vi "Previous VI.vi"(0 "PDF Report IN":refnum<class "PDF Report Class.lvclass">, 11 "error in (no error)":errorcluster) -> (4 "PDF Report OUT":refnum<class "PDF Report Class.lvclass">, 8 "Execute Actual VI":bool caption="实际执行 VI", 15 "error out":errorcluster)   [LabVIEW 2020, in "Exaprom PDF.lvlib"]
doc: "Version 1.0\nDeveloped by Jean-Marc Simard\nCopyright © 2010, Exaprom Inc.\nAll rights reserved.\nLicense: BSD\n\nWith iTextSharp 4.1.6 (http://itextsharp.sourceforge.net)\nunder Mozilla Public License Version 1.1\n(http://www.mozilla.org/MPL/MPL-1.1.html)"
uses:
  <userlib>/labview-PDF-writer-master/Exaprom PDF.lvlib
  <userlib>/labview-PDF-writer-master/LV Class/PDF Report Class/PDF Report Class.lvclass
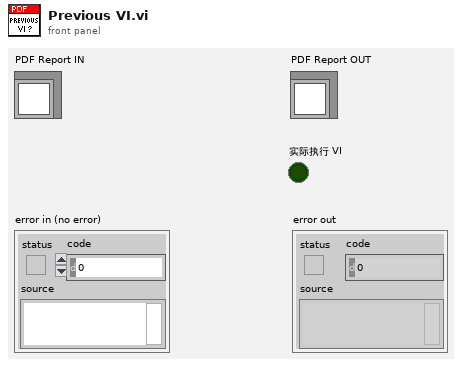
[diagram p1: front panel]
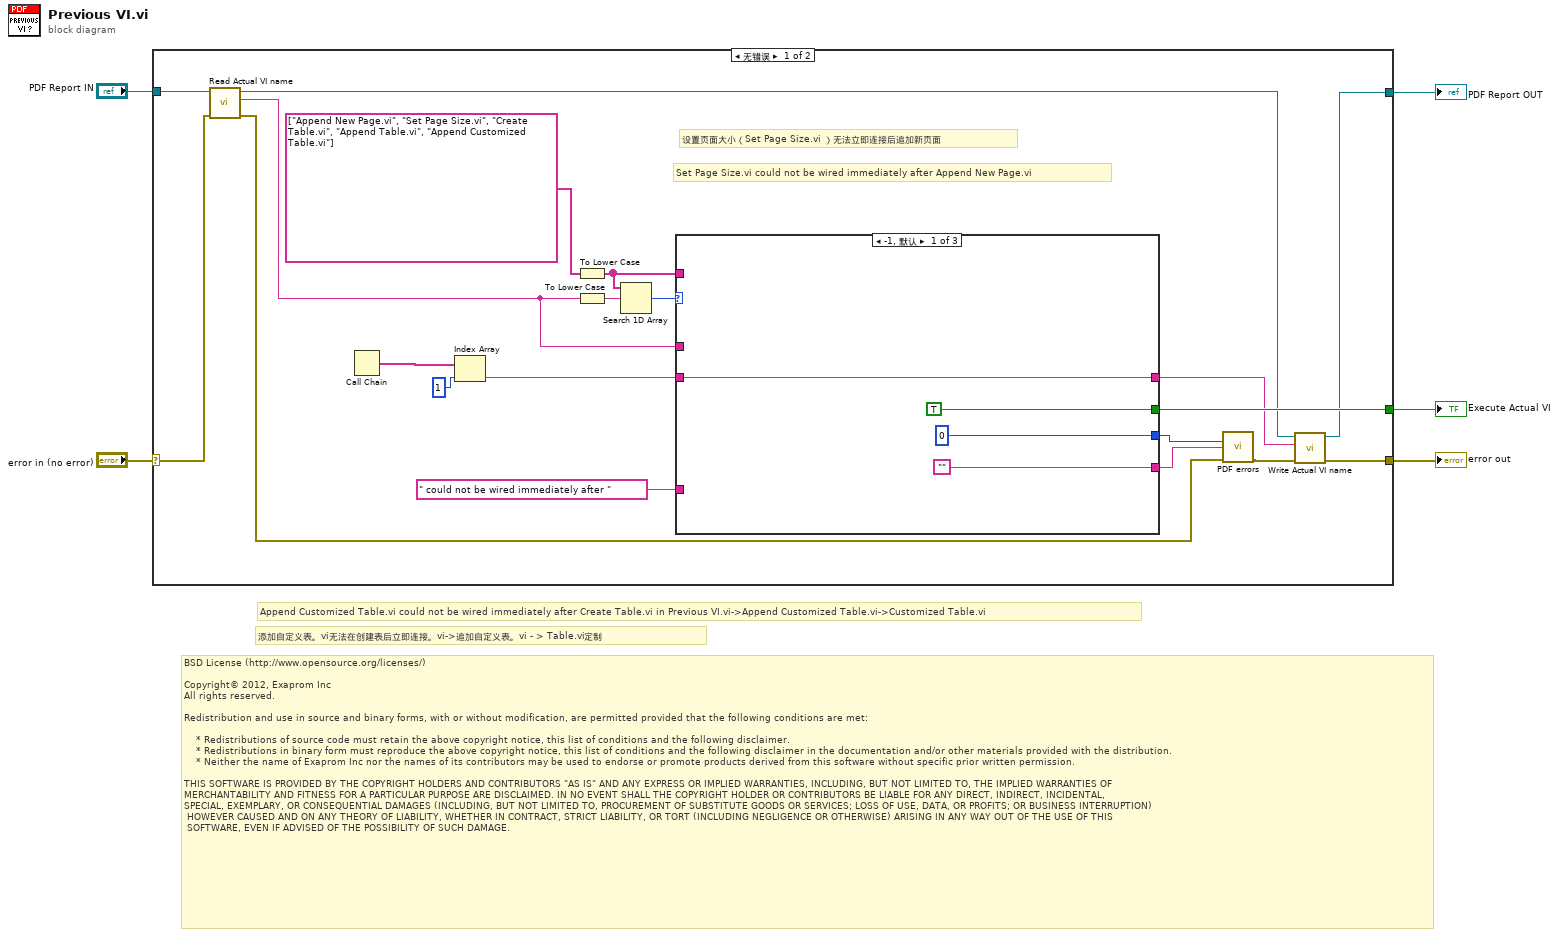
[diagram p0: block diagram]
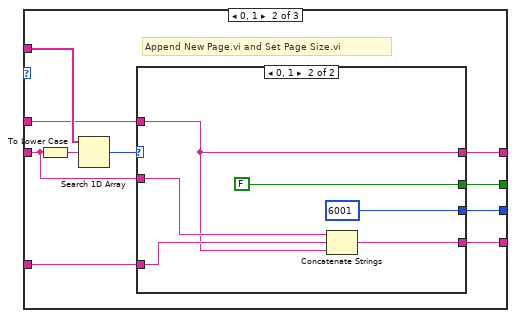
[diagram p2: hidden frame]
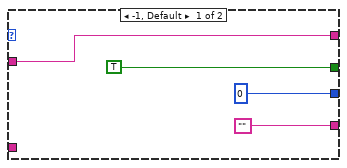
[diagram p3: hidden frame]
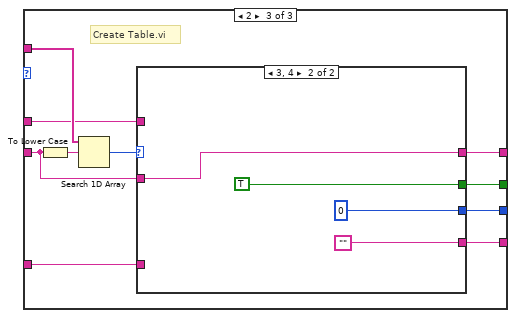
[diagram p4: hidden frame]
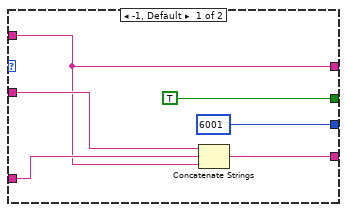
[diagram p5: hidden frame]
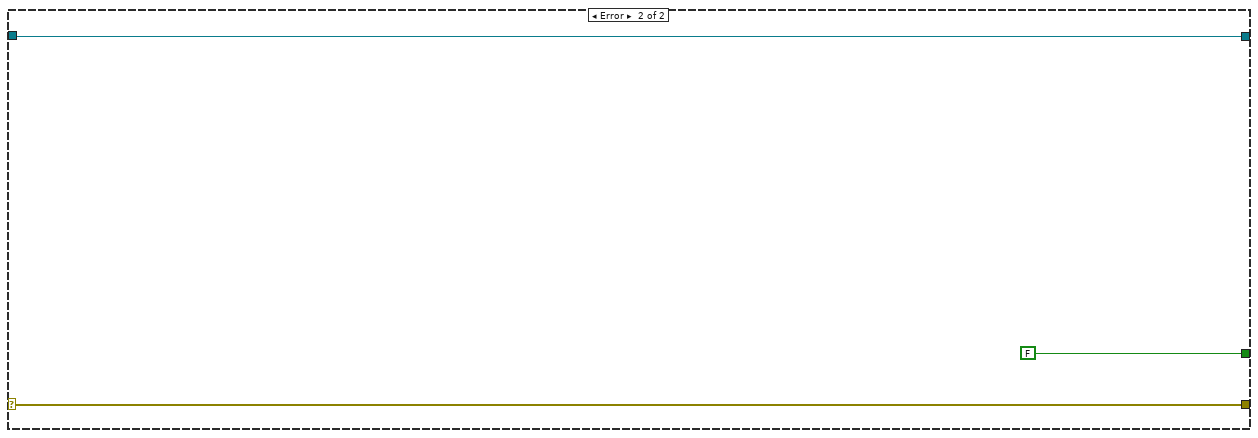
[diagram p6: hidden frame]
diagram:
  # "添加自定义表。vi无法在创建表后立即连接。vi->追加自定义表。vi - > Table.vi定制"
  # "Append Customized Table.vi could not be wired immediately after Create Table.vi in Previous VI.vi->Append Customized Table.vi->Customized Table.vi"
  # "BSD License (http://www.opensource.org/licenses/)\n\nCopyright© 2012, Exaprom Inc\nAll rights reserved.\n\nRedistribution and use in source and binary forms, with or without modification, are permitted provided that the following conditions are met:\n\n    * Redistributions of source code must retain the above copyright notice, this list of conditions and the following disclaimer.\n    * Redistributions in binary form must reproduce the above copyright notice, this list of conditions and the following disclaimer in the documentation and/or other materials provided with the distribution.\n    * Neither the name of Exaprom Inc nor the names of its contributors may be used to endorse or promote products derived from this software without specific prior written permission.\n\nTHIS SOFTWARE IS PROVIDED BY THE COPYRIGHT HOLDERS AND CONTRIBUTORS \"AS IS\" AND ANY EXPRESS OR IMPLIED WARRANTIES, INCLUDING, BUT NOT LIMITED TO, THE IMPLIED WARRANTIES OF \nMERCHANTABILITY AND FITNESS FOR A PARTICULAR PURPOSE ARE DISCLAIMED. IN NO EVENT SHALL THE COPYRIGHT HOLDER OR CONTRIBUTORS BE LIABLE FOR ANY DIRECT, INDIRECT, INCIDENTAL,\nSPECIAL, EXEMPLARY, OR CONSEQUENTIAL DAMAGES (INCLUDING, BUT NOT LIMITED TO, PROCUREMENT OF SUBSTITUTE GOODS OR SERVICES; LOSS OF USE, DATA, OR PROFITS; OR BUSINESS INTERRUPTION)\n HOWEVER CAUSED AND ON ANY THEORY OF LIABILITY, WHETHER IN CONTRACT, STRICT LIABILITY, OR TORT (INCLUDING NEGLIGENCE OR OTHERWISE) ARISING IN ANY WAY OUT OF THE USE OF THIS\n SOFTWARE, EVEN IF ADVISED OF THE POSSIBILITY OF SUCH DAMAGE."
  n1 = case shown="无错误" "error in (no error)" {
    selector: "error in (no error)" -> [w11 w72]
    tunnel: "PDF Report IN" -> [w13 w71]
    tunnel: [w6 w71] -> w4
    tunnel: [w9 w72] -> w3
    tunnel: [w15 FALSE] -> w1
    frame No Error {
      # "设置页面大小（Set Page Size.vi ）无法立即连接后追加新页面"
      # "Set Page Size.vi could not be wired immediately after Append New Page.vi"
      n2 = call-dynamic "Read Actual VI name.vi"("error in (no error)"=w11, "PDF Report Class in"=w13) -> ("error out"=w10:errorcluster, "Actual VI name"=w12:string, "PDF Report Class out"=w7:refnum<class "PDF Report Class.lvclass">)  [unwired: 7 in]
      n3 = Call Chain() -> (call chain=w23:string[])
      n4 = Index Array(array=w23, index=1) -> (element=w17:string)
      n5 = To Lower Case(string=string[] ["Append New Page.vi", "Set Page Size.vi", "Create Table.vi", "Append Table.vi", "Append Customized Table.vi"]) -> (all lower case string=w19:string[])
      n6 = To Lower Case(string=w12) -> (all lower case string=w24:string)
      n7 = Search 1D Array(1D array=w19, element=w24) -> (index of element=w18:i32)  [unwired: 1 out]
      n8 = case shown="-1, 默认" w18 {
        tunnel: w17 -> [w29 w35 w55]
        tunnel: w12 -> [_ w34 w54]
        tunnel: [w29 w36 w56] -> w8
        tunnel: w19 -> [_ w38 w58]
        tunnel: [TRUE w33 w53] -> w15
        tunnel: " could not be wired immediately after " -> [_ w32 w52]
        tunnel: ["" w31 w50] -> w21
        tunnel: [0 ("y") w30 w51] -> w20
        frame -1, Default {
        }
        frame 0, 1 {
          # "Append New Page.vi and Set Page Size.vi"
          n9 = To Lower Case(string=w35) -> (all lower case string=w39:string)
          n10 = Search 1D Array(1D array=w38, element=w39) -> (index of element=w37:i32)  [unwired: 1 out]
          n11 = case shown="0, 1" w37 {
            tunnel: [w43 w46] -> w36
            tunnel: w35 -> [w43 w47]
            tunnel: w34 -> [_ w46]
            tunnel: [TRUE FALSE] -> w33
            tunnel: w32 -> [_ w48]
            tunnel: ["" w45] -> w31
            tunnel: [0 ("y") 6001 ("y")] -> w30
            frame -1, Default {
            }
            frame 0, 1 {
              n12 = Concatenate Strings(w47, w48, w46) -> (w45:string)
            }
          }
        }
        frame 2 {
          # "Create Table.vi"
          n13 = To Lower Case(string=w55) -> (all lower case string=w59:string)
          n14 = Search 1D Array(1D array=w58, element=w59) -> (index of element=w57:i32)  [unwired: 1 out]
          n15 = case shown="3, 4" w57 {
            tunnel: [w62 w68] -> w56
            tunnel: w55 -> [w63 w68]
            tunnel: w54 -> [w62 _]
            tunnel: [TRUE TRUE] -> w53
            tunnel: w52 -> [w64 _]
            tunnel: [6001 ("y") 0 ("y")] -> w51
            tunnel: [w61 ""] -> w50
            frame -1, Default {
              n16 = Concatenate Strings(w63, w64, w62) -> (w61:string)
            }
            frame 3, 4 {
            }
          }
        }
      }
      n17 = call <userlib>:"PDF errors.vi"("code"=w20, "Additionnal information"=w21, "error in (no error)"=w10) -> ("error out"=w14:errorcluster)  [unwired: 12 out]
      n18 = call-dynamic "Write Actual VI name.vi"("error in (no error)"=w14, "Actual VI name"=w8, "PDF Report Class in"=w7) -> ("error out"=w9:errorcluster, "PDF Report Class out"=w6:refnum<class "PDF Report Class.lvclass">)  [unwired: 7 in]
    }
    frame Error {
    }
  }
  "PDF Report OUT" <- w4
  "error out" <- w3
  "Execute Actual VI" <- w1
